vi "Get Node Attribute Value.vi"(10 "Attribute Name":string, 11 "Refnum in":refnum<k20>) -> (3 "Value":string)   [LabVIEW 2025]
uses:
  <resource>/objmgr/DOMUserDefRef.rc
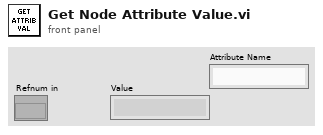
[diagram p1: front panel]
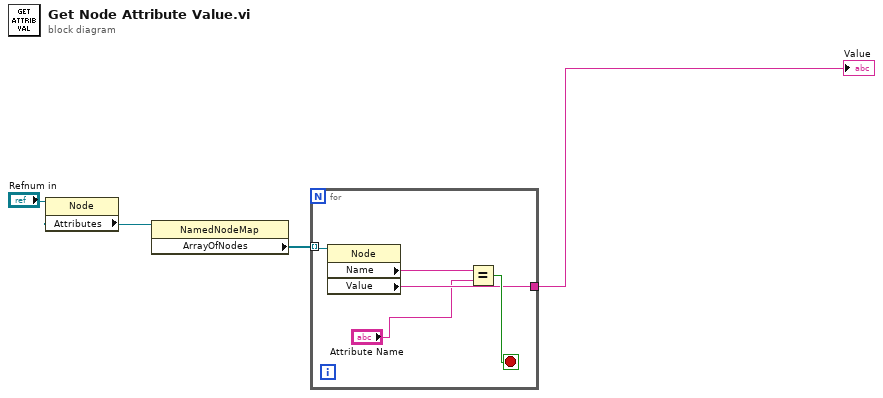
[diagram p0: block diagram]
diagram:
  n1 = property class="Node"(reference="Refnum in") -> ("Attributes"=w2:refnum<k20>)  [unwired: 1 in, 2 out]
  n2 = property class="NamedNodeMap"(reference=w2) -> ("ArrayOfNodes"=w3:refnum<k20>[])  [unwired: 1 in, 2 out]
  n3 = for {
    tunnel: w3 -> [w9] mode=indexing
    tunnel: [w6] -> w4
    stop <- w7 stop-if-true
    n4 = property class="Node"(reference=w9) -> ("Name"=w8:string, "Value"=w6:string)  [unwired: 1 in, 2 out]
    n5 = Equal?(x=w8, y="Attribute Name") -> (x = y?=w7:bool)
  }
  "Value" <- w4
